vi "数字量输出配置.vi"() -> ()   [LabVIEW 2010] (continued)
              tunnel: [FALSE ("单选_第41路") TRUE ("单选_第41路")] -> w551
              frame False {
              }
              frame True {
              }
            }
            n6526 = local write "单选_第49路"(w551) -> ()
            n6527 = local write "单选_第50路"(w551) -> ()
            n6528 = local write "单选_第51路"(w551) -> ()
            n6529 = local write "单选_第52路"(w551) -> ()
            n6530 = local write "单选_第53路"(w551) -> ()
            n6531 = local write "单选_第54路"(w551) -> ()
            n6532 = local write "单选_第55路"(w551) -> ()
            n6533 = local write "单选_第56路"(w551) -> ()
            n6534 = local write "单选_第57路"(w551) -> ()
            n6535 = local write "单选_第58路"(w551) -> ()
            n6536 = local write "单选_第59路"(w551) -> ()
            n6537 = local write "单选_第60路"(w551) -> ()
            n6538 = local write "单选_第61路"(w551) -> ()
            n6539 = local write "单选_第62路"(w551) -> ()
            n6540 = local write "单选_第63路"(w551) -> ()
            n6541 = local write "单选_第64路"(w551) -> ()
          }
          event "btn_全选_5": Value Change {
            n6542 = event-data() -> ("NewVal"=w556:bool)  [unwired: 1 in, 4 out]
            n6543 = case shown="假" w556 {
              tunnel: [FALSE ("单选_第41路") TRUE ("单选_第41路")] -> w555
              frame False {
              }
              frame True {
              }
            }
            n6544 = local write "单选_第71路"(w555) -> ()
            n6545 = local write "单选_第79路"(w555) -> ()
            n6546 = local write "单选_第65路"(w555) -> ()
            n6547 = local write "单选_第66路"(w555) -> ()
            n6548 = local write "单选_第67路"(w555) -> ()
            n6549 = local write "单选_第68路"(w555) -> ()
            n6550 = local write "单选_第69路"(w555) -> ()
            n6551 = local write "单选_第70路"(w555) -> ()
            n6552 = local write "单选_第72路"(w555) -> ()
            n6553 = local write "单选_第73路"(w555) -> ()
            n6554 = local write "单选_第74路"(w555) -> ()
            n6555 = local write "单选_第75路"(w555) -> ()
            n6556 = local write "单选_第76路"(w555) -> ()
            n6557 = local write "单选_第77路"(w555) -> ()
            n6558 = local write "单选_第78路"(w555) -> ()
            n6559 = local write "单选_第80路"(w555) -> ()
          }
          event "btn_置1_1": Value Change {
            n6560 = event-data() -> ("NewVal"=w560:bool)  [unwired: 1 in, 4 out]
            n6561 = case shown="假" w560 {
              tunnel: [enum16{"0", "1"}."0" ("输入值_41") enum16{"0", "1"}."1" ("输入值_41")] -> w559
              frame False {
              }
              frame True {
              }
            }
            n6562 = local write "输入值_1"(w559) -> ()
            n6563 = local write "输入值_2"(w559) -> ()
            n6564 = local write "输入值_3"(w559) -> ()
            n6565 = local write "输入值_4"(w559) -> ()
            n6566 = local write "输入值_5"(w559) -> ()
            n6567 = local write "输入值_6"(w559) -> ()
            n6568 = local write "输入值_7"(w559) -> ()
            n6569 = local write "输入值_8"(w559) -> ()
            n6570 = local write "输入值_9"(w559) -> ()
            n6571 = local write "输入值_10"(w559) -> ()
            n6572 = local write "输入值_11"(w559) -> ()
            n6573 = local write "输入值_12"(w559) -> ()
            n6574 = local write "输入值_13"(w559) -> ()
            n6575 = local write "输入值_14"(w559) -> ()
            n6576 = local write "输入值_15"(w559) -> ()
            n6577 = local write "输入值_16"(w559) -> ()
          }
          event "btn_置1_2": Value Change {
            n6578 = event-data() -> ("NewVal"=w564:bool)  [unwired: 1 in, 4 out]
            n6579 = case shown="假" w564 {
              tunnel: [enum16{"0", "1"}."0" ("输入值_41") enum16{"0", "1"}."1" ("输入值_41")] -> w563
              frame False {
              }
              frame True {
              }
            }
            n6580 = local write "输入值_17"(w563) -> ()
            n6581 = local write "输入值_18"(w563) -> ()
            n6582 = local write "输入值_19"(w563) -> ()
            n6583 = local write "输入值_20"(w563) -> ()
            n6584 = local write "输入值_21"(w563) -> ()
            n6585 = local write "输入值_22"(w563) -> ()
            n6586 = local write "输入值_23"(w563) -> ()
            n6587 = local write "输入值_24"(w563) -> ()
            n6588 = local write "输入值_25"(w563) -> ()
            n6589 = local write "输入值_26"(w563) -> ()
            n6590 = local write "输入值_27"(w563) -> ()
            n6591 = local write "输入值_28"(w563) -> ()
            n6592 = local write "输入值_29"(w563) -> ()
            n6593 = local write "输入值_30"(w563) -> ()
            n6594 = local write "输入值_31"(w563) -> ()
            n6595 = local write "输入值_32"(w563) -> ()
          }
          event "btn_置1_3": Value Change {
            n6596 = event-data() -> ("NewVal"=w568:bool)  [unwired: 1 in, 4 out]
            n6597 = case shown="假" w568 {
              tunnel: [enum16{"0", "1"}."0" ("输入值_41") enum16{"0", "1"}."1" ("输入值_41")] -> w567
              frame False {
              }
              frame True {
              }
            }
            n6598 = local write "输入值_33"(w567) -> ()
            n6599 = local write "输入值_34"(w567) -> ()
            n6600 = local write "输入值_35"(w567) -> ()
            n6601 = local write "输入值_36"(w567) -> ()
            n6602 = local write "输入值_37"(w567) -> ()
            n6603 = local write "输入值_38"(w567) -> ()
            n6604 = local write "输入值_39"(w567) -> ()
            n6605 = local write "输入值_40"(w567) -> ()
            n6606 = local write "输入值_41"(w567) -> ()
            n6607 = local write "输入值_42"(w567) -> ()
            n6608 = local write "输入值_43"(w567) -> ()
            n6609 = local write "输入值_44"(w567) -> ()
            n6610 = local write "输入值_45"(w567) -> ()
            n6611 = local write "输入值_46"(w567) -> ()
            n6612 = local write "输入值_47"(w567) -> ()
            n6613 = local write "输入值_48"(w567) -> ()
          }
          event "btn_置1_4": Value Change {
            n6614 = event-data() -> ("NewVal"=w572:bool)  [unwired: 1 in, 4 out]
            n6615 = case shown="假" w572 {
              tunnel: [enum16{"0", "1"}."0" ("输入值_41") enum16{"0", "1"}."1" ("输入值_41")] -> w571
              frame False {
              }
              frame True {
              }
            }
            n6616 = local write "输入值_49"(w571) -> ()
            n6617 = local write "输入值_50"(w571) -> ()
            n6618 = local write "输入值_51"(w571) -> ()
            n6619 = local write "输入值_52"(w571) -> ()
            n6620 = local write "输入值_53"(w571) -> ()
            n6621 = local write "输入值_54"(w571) -> ()
            n6622 = local write "输入值_55"(w571) -> ()
            n6623 = local write "输入值_56"(w571) -> ()
            n6624 = local write "输入值_57"(w571) -> ()
            n6625 = local write "输入值_58"(w571) -> ()
            n6626 = local write "输入值_59"(w571) -> ()
            n6627 = local write "输入值_60"(w571) -> ()
            n6628 = local write "输入值_61"(w571) -> ()
            n6629 = local write "输入值_62"(w571) -> ()
            n6630 = local write "输入值_63"(w571) -> ()
            n6631 = local write "输入值_64"(w571) -> ()
          }
          event "btn_置1_5": Value Change {
            n6632 = event-data() -> ("NewVal"=w576:bool)  [unwired: 1 in, 4 out]
            n6633 = case shown="假" w576 {
              tunnel: [enum16{"0", "1"}."0" ("输入值_41") enum16{"0", "1"}."1" ("输入值_41")] -> w575
              frame False {
              }
              frame True {
              }
            }
            n6634 = local write "输入值_65"(w575) -> ()
            n6635 = local write "输入值_66"(w575) -> ()
            n6636 = local write "输入值_67"(w575) -> ()
            n6637 = local write "输入值_68"(w575) -> ()
            n6638 = local write "输入值_69"(w575) -> ()
            n6639 = local write "输入值_70"(w575) -> ()
            n6640 = local write "输入值_71"(w575) -> ()
            n6641 = local write "输入值_72"(w575) -> ()
            n6642 = local write "输入值_73"(w575) -> ()
            n6643 = local write "输入值_74"(w575) -> ()
            n6644 = local write "输入值_75"(w575) -> ()
            n6645 = local write "输入值_76"(w575) -> ()
            n6646 = local write "输入值_77"(w575) -> ()
            n6647 = local write "输入值_78"(w575) -> ()
            n6648 = local write "输入值_79"(w575) -> ()
            n6649 = local write "输入值_80"(w575) -> ()
          }
          event "btn_开始试验": Value Change {
            n6650 = event-data() -> ()  [unwired: 1 in, 5 out]
            n6651 = stacked-sequence {
              frame #0 {
                w580 = 0 ("同步_A1")
                n6652 = stacked-sequence {
                  tunnel: [w606 _ _ _ _] -> w602
                  tunnel: [w605 _ _ _ _] -> w586
                  tunnel: [_ w640 _ _ _] -> w600
                  tunnel: [_ w639 _ _ _] -> w585
                  tunnel: [_ _ w674 _ _] -> w598
                  tunnel: [_ _ w673 _ _] -> w584
                  tunnel: [_ _ _ w708 _] -> w596
                  tunnel: [_ _ _ w707 _] -> w583
                  tunnel: [_ _ _ _ w742] -> w594
                  tunnel: [_ _ _ _ w741] -> w582
                  frame #0 {
                    n6653 = local read "单选_第1路"() -> (w623:bool)
                    n6654 = local read "单选_第2路"() -> (w624:bool)
                    n6655 = local read "单选_第3路"() -> (w625:bool)
                    n6656 = local read "单选_第4路"() -> (w626:bool)
                    n6657 = local read "单选_第5路"() -> (w627:bool)
                    n6658 = local read "单选_第6路"() -> (w628:bool)
                    n6659 = local read "单选_第7路"() -> (w629:bool)
                    n6660 = local read "单选_第8路"() -> (w630:bool)
                    n6661 = local read "单选_第9路"() -> (w631:bool)
                    n6662 = local read "单选_第10路"() -> (w632:bool)
                    n6663 = local read "单选_第11路"() -> (w633:bool)
                    n6664 = local read "单选_第12路"() -> (w634:bool)
                    n6665 = local read "单选_第13路"() -> (w635:bool)
                    n6666 = local read "单选_第14路"() -> (w636:bool)
                    n6667 = local read "单选_第15路"() -> (w637:bool)
                    n6668 = local read "单选_第16路"() -> (w638:bool)
                    n6669 = local read "输入值_1"() -> (w607:enum16{"0", "1"})
                    n6670 = local read "输入值_2"() -> (w608:enum16{"0", "1"})
                    n6671 = local read "输入值_3"() -> (w609:enum16{"0", "1"})
                    n6672 = local read "输入值_4"() -> (w610:enum16{"0", "1"})
                    n6673 = local read "输入值_5"() -> (w611:enum16{"0", "1"})
                    n6674 = local read "输入值_6"() -> (w612:enum16{"0", "1"})
                    n6675 = local read "输入值_7"() -> (w613:enum16{"0", "1"})
                    n6676 = local read "输入值_8"() -> (w614:enum16{"0", "1"})
                    n6677 = local read "输入值_9"() -> (w615:enum16{"0", "1"})
                    n6678 = local read "输入值_10"() -> (w616:enum16{"0", "1"})
                    n6679 = local read "输入值_11"() -> (w617:enum16{"0", "1"})
                    n6680 = local read "输入值_12"() -> (w618:enum16{"0", "1"})
                    n6681 = local read "输入值_13"() -> (w619:enum16{"0", "1"})
                    n6682 = local read "输入值_14"() -> (w620:enum16{"0", "1"})
                    n6683 = local read "输入值_15"() -> (w621:enum16{"0", "1"})
                    n6684 = local read "输入值_16"() -> (w622:enum16{"0", "1"})
                    n6685 = Build Array(w623, w624, w625, w626, w627, w628, w629, w630, w631, w632, w633, w634, w635, w636, w637, w638) -> (w606:bool[])
                    n6686 = Build Array(w607, w608, w609, w610, w611, w612, w613, w614, w615, w616, w617, w618, w619, w620, w621, w622) -> (w605:enum16{"0", "1"}[])
                  }
                  frame #1 {
                    n6687 = local read "单选_第17路"() -> (w657:bool)
                    n6688 = local read "单选_第18路"() -> (w658:bool)
                    n6689 = local read "单选_第19路"() -> (w659:bool)
                    n6690 = local read "单选_第20路"() -> (w660:bool)
                    n6691 = local read "单选_第21路"() -> (w661:bool)
                    n6692 = local read "单选_第22路"() -> (w662:bool)
                    n6693 = local read "单选_第23路"() -> (w663:bool)
                    n6694 = local read "单选_第24路"() -> (w664:bool)
                    n6695 = local read "单选_第25路"() -> (w665:bool)
                    n6696 = local read "单选_第26路"() -> (w666:bool)
                    n6697 = local read "单选_第27路"() -> (w667:bool)
                    n6698 = local read "单选_第28路"() -> (w668:bool)
                    n6699 = local read "单选_第29路"() -> (w669:bool)
                    n6700 = local read "单选_第30路"() -> (w670:bool)
                    n6701 = local read "单选_第31路"() -> (w671:bool)
                    n6702 = local read "单选_第32路"() -> (w672:bool)
                    n6703 = local read "输入值_17"() -> (w641:enum16{"0", "1"})
                    n6704 = local read "输入值_18"() -> (w642:enum16{"0", "1"})
                    n6705 = local read "输入值_19"() -> (w643:enum16{"0", "1"})
                    n6706 = local read "输入值_20"() -> (w644:enum16{"0", "1"})
                    n6707 = local read "输入值_21"() -> (w645:enum16{"0", "1"})
                    n6708 = local read "输入值_22"() -> (w646:enum16{"0", "1"})
                    n6709 = local read "输入值_23"() -> (w647:enum16{"0", "1"})
                    n6710 = local read "输入值_24"() -> (w648:enum16{"0", "1"})
                    n6711 = local read "输入值_25"() -> (w649:enum16{"0", "1"})
                    n6712 = local read "输入值_26"() -> (w650:enum16{"0", "1"})
                    n6713 = local read "输入值_27"() -> (w651:enum16{"0", "1"})
                    n6714 = local read "输入值_28"() -> (w652:enum16{"0", "1"})
                    n6715 = local read "输入值_29"() -> (w653:enum16{"0", "1"})
                    n6716 = local read "输入值_30"() -> (w654:enum16{"0", "1"})
                    n6717 = local read "输入值_31"() -> (w655:enum16{"0", "1"})
                    n6718 = local read "输入值_32"() -> (w656:enum16{"0", "1"})
                    n6719 = Build Array(w657, w658, w659, w660, w661, w662, w663, w664, w665, w666, w667, w668, w669, w670, w671, w672) -> (w640:bool[])
                    n6720 = Build Array(w641, w642, w643, w644, w645, w646, w647, w648, w649, w650, w651, w652, w653, w654, w655, w656) -> (w639:enum16{"0", "1"}[])
                  }
                  frame #2 {
                    n6721 = local read "单选_第33路"() -> (w691:bool)
                    n6722 = local read "单选_第34路"() -> (w692:bool)
                    n6723 = local read "单选_第35路"() -> (w693:bool)
                    n6724 = local read "单选_第36路"() -> (w694:bool)
                    n6725 = local read "单选_第37路"() -> (w695:bool)
                    n6726 = local read "单选_第38路"() -> (w696:bool)
                    n6727 = local read "单选_第39路"() -> (w697:bool)
                    n6728 = local read "单选_第40路"() -> (w698:bool)
                    n6729 = local read "单选_第41路"() -> (w699:bool)
                    n6730 = local read "单选_第42路"() -> (w700:bool)
                    n6731 = local read "单选_第43路"() -> (w701:bool)
                    n6732 = local read "单选_第44路"() -> (w702:bool)
                    n6733 = local read "单选_第45路"() -> (w703:bool)
                    n6734 = local read "单选_第46路"() -> (w704:bool)
                    n6735 = local read "单选_第47路"() -> (w705:bool)
                    n6736 = local read "单选_第48路"() -> (w706:bool)
                    n6737 = local read "输入值_33"() -> (w675:enum16{"0", "1"})
                    n6738 = local read "输入值_34"() -> (w676:enum16{"0", "1"})
                    n6739 = local read "输入值_35"() -> (w677:enum16{"0", "1"})
                    n6740 = local read "输入值_36"() -> (w678:enum16{"0", "1"})
                    n6741 = local read "输入值_37"() -> (w679:enum16{"0", "1"})
                    n6742 = local read "输入值_38"() -> (w680:enum16{"0", "1"})
                    n6743 = local read "输入值_39"() -> (w681:enum16{"0", "1"})
                    n6744 = local read "输入值_40"() -> (w682:enum16{"0", "1"})
                    n6745 = local read "输入值_41"() -> (w683:enum16{"0", "1"})
                    n6746 = local read "输入值_42"() -> (w684:enum16{"0", "1"})
                    n6747 = local read "输入值_43"() -> (w685:enum16{"0", "1"})
                    n6748 = local read "输入值_44"() -> (w686:enum16{"0", "1"})
                    n6749 = local read "输入值_45"() -> (w687:enum16{"0", "1"})
                    n6750 = local read "输入值_46"() -> (w688:enum16{"0", "1"})
                    n6751 = local read "输入值_47"() -> (w689:enum16{"0", "1"})
                    n6752 = local read "输入值_48"() -> (w690:enum16{"0", "1"})
                    n6753 = Build Array(w675, w676, w677, w678, w679, w680, w681, w682, w683, w684, w685, w686, w687, w688, w689, w690) -> (w673:enum16{"0", "1"}[])
                    n6754 = Build Array(w691, w692, w693, w694, w695, w696, w697, w698, w699, w700, w701, w702, w703, w704, w705, w706) -> (w674:bool[])
                  }
                  frame #3 {
                    n6755 = local read "单选_第49路"() -> (w725:bool)
                    n6756 = local read "单选_第50路"() -> (w726:bool)
                    n6757 = local read "单选_第51路"() -> (w727:bool)
                    n6758 = local read "单选_第52路"() -> (w728:bool)
                    n6759 = local read "单选_第53路"() -> (w729:bool)
                    n6760 = local read "单选_第54路"() -> (w730:bool)
                    n6761 = local read "单选_第55路"() -> (w731:bool)
                    n6762 = local read "单选_第56路"() -> (w732:bool)
                    n6763 = local read "单选_第57路"() -> (w733:bool)
                    n6764 = local read "单选_第58路"() -> (w734:bool)
                    n6765 = local read "单选_第59路"() -> (w735:bool)
                    n6766 = local read "单选_第60路"() -> (w736:bool)
                    n6767 = local read "单选_第61路"() -> (w737:bool)
                    n6768 = local read "单选_第62路"() -> (w738:bool)
                    n6769 = local read "单选_第63路"() -> (w739:bool)
                    n6770 = local read "单选_第64路"() -> (w740:bool)
                    n6771 = local read "输入值_49"() -> (w709:enum16{"0", "1"})
                    n6772 = local read "输入值_50"() -> (w710:enum16{"0", "1"})
                    n6773 = local read "输入值_51"() -> (w711:enum16{"0", "1"})
                    n6774 = local read "输入值_52"() -> (w712:enum16{"0", "1"})
                    n6775 = local read "输入值_53"() -> (w713:enum16{"0", "1"})
                    n6776 = local read "输入值_54"() -> (w714:enum16{"0", "1"})
                    n6777 = local read "输入值_55"() -> (w715:enum16{"0", "1"})
                    n6778 = local read "输入值_56"() -> (w716:enum16{"0", "1"})
                    n6779 = local read "输入值_57"() -> (w717:enum16{"0", "1"})
                    n6780 = local read "输入值_58"() -> (w718:enum16{"0", "1"})
                    n6781 = local read "输入值_59"() -> (w719:enum16{"0", "1"})
                    n6782 = local read "输入值_60"() -> (w720:enum16{"0", "1"})
                    n6783 = local read "输入值_61"() -> (w721:enum16{"0", "1"})
                    n6784 = local read "输入值_62"() -> (w722:enum16{"0", "1"})
                    n6785 = local read "输入值_63"() -> (w723:enum16{"0", "1"})
                    n6786 = local read "输入值_64"() -> (w724:enum16{"0", "1"})
                    n6787 = Build Array(w725, w726, w727, w728, w729, w730, w731, w732, w733, w734, w735, w736, w737, w738, w739, w740) -> (w708:bool[])
                    n6788 = Build Array(w709, w710, w711, w712, w713, w714, w715, w716, w717, w718, w719, w720, w721, w722, w723, w724) -> (w707:enum16{"0", "1"}[])
                  }
                  frame #4 {
                    n6789 = local read "单选_第71路"() -> (w765:bool)
                    n6790 = local read "单选_第79路"() -> (w773:bool)
                    n6791 = local read "单选_第65路"() -> (w759:bool)
                    n6792 = local read "单选_第66路"() -> (w760:bool)
                    n6793 = local read "单选_第67路"() -> (w761:bool)
                    n6794 = local read "单选_第68路"() -> (w762:bool)
                    n6795 = local read "单选_第69路"() -> (w763:bool)
                    n6796 = local read "单选_第70路"() -> (w764:bool)
                    n6797 = local read "单选_第72路"() -> (w766:bool)
                    n6798 = local read "单选_第73路"() -> (w767:bool)
                    n6799 = local read "单选_第74路"() -> (w768:bool)
                    n6800 = local read "单选_第75路"() -> (w769:bool)
                    n6801 = local read "单选_第76路"() -> (w770:bool)
                    n6802 = local read "单选_第77路"() -> (w771:bool)
                    n6803 = local read "单选_第78路"() -> (w772:bool)
                    n6804 = local read "单选_第80路"() -> (w774:bool)
                    n6805 = local read "输入值_65"() -> (w743:enum16{"0", "1"})
                    n6806 = local read "输入值_66"() -> (w744:enum16{"0", "1"})
                    n6807 = local read "输入值_67"() -> (w745:enum16{"0", "1"})
                    n6808 = local read "输入值_68"() -> (w746:enum16{"0", "1"})
                    n6809 = local read "输入值_69"() -> (w747:enum16{"0", "1"})
                    n6810 = local read "输入值_70"() -> (w748:enum16{"0", "1"})
                    n6811 = local read "输入值_71"() -> (w749:enum16{"0", "1"})
                    n6812 = local read "输入值_72"() -> (w750:enum16{"0", "1"})
                    n6813 = local read "输入值_73"() -> (w751:enum16{"0", "1"})
                    n6814 = local read "输入值_74"() -> (w752:enum16{"0", "1"})
                    n6815 = local read "输入值_75"() -> (w753:enum16{"0", "1"})
                    n6816 = local read "输入值_76"() -> (w754:enum16{"0", "1"})
                    n6817 = local read "输入值_77"() -> (w755:enum16{"0", "1"})
                    n6818 = local read "输入值_78"() -> (w756:enum16{"0", "1"})
                    n6819 = local read "输入值_79"() -> (w757:enum16{"0", "1"})
                    n6820 = local read "输入值_80"() -> (w758:enum16{"0", "1"})
                    n6821 = Build Array(w743, w744, w745, w746, w747, w748, w749, w750, w751, w752, w753, w754, w755, w756, w757, w758) -> (w741:enum16{"0", "1"}[])
                    n6822 = Build Array(w759, w760, w761, w762, w763, w764, w765, w766, w767, w768, w769, w770, w771, w772, w773, w774) -> (w742:bool[])
                  }
                }
                n6823 = local read "数组_选择?"() -> (w604:bool[][])
                n6824 = local read "数组_输入值"() -> (w587:enum16{"0", "1"}[][])
                n6825 = Replace Array Subset(array=w604, new element #1=w602, index (row) #1=0 ("索引 (行)"), new element #2=w600, index (row) #2=1 ("索引 (行)"), new element #3=w598, index (row) #3=2 ("索引 (行)"), new element #4=w596, index (row) #4=3 ("索引 (行)"), new element #5=w594, index (row) #5=4 ("索引 (行)")) -> (w593:bool[][])  [unwired: 5 in]
                n6826 = local write "测试结论"("") -> ()
                n6827 = local write "同步_A1"(w580) -> ()
                n6828 = local write "同步_A2"(w580) -> ()
                n6829 = Replace Array Subset(array=w587, new element #1=w586, index (row) #1=0 ("索引 (行)"), new element #2=w585, index (row) #2=1 ("索引 (行)"), new element #3=w584, index (row) #3=2 ("索引 (行)"), new element #4=w583, index (row) #4=3 ("索引 (行)"), new element #5=w582, index (row) #5=4 ("索引 (行)")) -> (w581:enum16{"0", "1"}[][])  [unwired: 5 in]
                n6830 = local write "数组_输入值"(w581) -> ()
                n6831 = local write "数组_选择?"(w593) -> ()
              }
              frame #1 {
                w775 = cluster{u32, u32}[] [{9868950, 9868950}]
                n6832 = property on="light_1" class="Bool (严格)"("Colors [4]"=w775) -> ()  [unwired: 2 in, 2 out]
                n6833 = property on="light_2" class="Bool (严格)"("Colors [4]"=w775) -> ()  [unwired: 2 in, 2 out]
                n6834 = property on="light_3" class="Bool (严格)"("Colors [4]"=w775) -> ()  [unwired: 2 in, 2 out]
                n6835 = property on="light_4" class="Bool (严格)"("Colors [4]"=w775) -> ()  [unwired: 2 in, 2 out]
                n6836 = property on="light_5" class="Bool (严格)"("Colors [4]"=w775) -> ()  [unwired: 2 in, 2 out]
                n6837 = property on="light_6" class="Bool (严格)"("Colors [4]"=w775) -> ()  [unwired: 2 in, 2 out]
                n6838 = property on="light_7" class="Bool (严格)"("Colors [4]"=w775) -> ()  [unwired: 2 in, 2 out]
                n6839 = property on="light_8" class="Bool (严格)"("Colors [4]"=w775) -> ()  [unwired: 2 in, 2 out]
                n6840 = property on="light_9" class="Bool (严格)"("Colors [4]"=w775) -> ()  [unwired: 2 in, 2 out]
                n6841 = property on="light_10" class="Bool (严格)"("Colors [4]"=w775) -> ()  [unwired: 2 in, 2 out]
                n6842 = property on="light_11" class="Bool (严格)"("Colors [4]"=w775) -> ()  [unwired: 2 in, 2 out]
                n6843 = property on="light_12" class="Bool (严格)"("Colors [4]"=w775) -> ()  [unwired: 2 in, 2 out]
                n6844 = property on="light_13" class="Bool (严格)"("Colors [4]"=w775) -> ()  [unwired: 2 in, 2 out]
                n6845 = property on="light_14" class="Bool (严格)"("Colors [4]"=w775) -> ()  [unwired: 2 in, 2 out]
                n6846 = property on="light_15" class="Bool (严格)"("Colors [4]"=w775) -> ()  [unwired: 2 in, 2 out]
                n6847 = property on="light_16" class="Bool (严格)"("Colors [4]"=w775) -> ()  [unwired: 2 in, 2 out]
                n6848 = property on="light_17" class="Bool (严格)"("Colors [4]"=w775) -> ()  [unwired: 2 in, 2 out]
                n6849 = property on="light_18" class="Bool (严格)"("Colors [4]"=w775) -> ()  [unwired: 2 in, 2 out]
                n6850 = property on="light_19" class="Bool (严格)"("Colors [4]"=w775) -> ()  [unwired: 2 in, 2 out]
                n6851 = property on="light_20" class="Bool (严格)"("Colors [4]"=w775) -> ()  [unwired: 2 in, 2 out]
                n6852 = property on="light_21" class="Bool (严格)"("Colors [4]"=w775) -> ()  [unwired: 2 in, 2 out]
                n6853 = property on="light_22" class="Bool (严格)"("Colors [4]"=w775) -> ()  [unwired: 2 in, 2 out]
                n6854 = property on="light_23" class="Bool (严格)"("Colors [4]"=w775) -> ()  [unwired: 2 in, 2 out]
                n6855 = property on="light_24" class="Bool (严格)"("Colors [4]"=w775) -> ()  [unwired: 2 in, 2 out]
                n6856 = property on="light_25" class="Bool (严格)"("Colors [4]"=w775) -> ()  [unwired: 2 in, 2 out]
                n6857 = property on="light_26" class="Bool (严格)"("Colors [4]"=w775) -> ()  [unwired: 2 in, 2 out]
                n6858 = property on="light_27" class="Bool (严格)"("Colors [4]"=w775) -> ()  [unwired: 2 in, 2 out]
                n6859 = property on="light_28" class="Bool (严格)"("Colors [4]"=w775) -> ()  [unwired: 2 in, 2 out]
                n6860 = property on="light_29" class="Bool (严格)"("Colors [4]"=w775) -> ()  [unwired: 2 in, 2 out]
                n6861 = property on="light_30" class="Bool (严格)"("Colors [4]"=w775) -> ()  [unwired: 2 in, 2 out]
                n6862 = property on="light_31" class="Bool (严格)"("Colors [4]"=w775) -> ()  [unwired: 2 in, 2 out]
                n6863 = property on="light_32" class="Bool (严格)"("Colors [4]"=w775) -> ()  [unwired: 2 in, 2 out]
                n6864 = property on="light_33" class="Bool (严格)"("Colors [4]"=w775) -> ()  [unwired: 2 in, 2 out]
                n6865 = property on="light_34" class="Bool (严格)"("Colors [4]"=w775) -> ()  [unwired: 2 in, 2 out]
                n6866 = property on="light_35" class="Bool (严格)"("Colors [4]"=w775) -> ()  [unwired: 2 in, 2 out]
                n6867 = property on="light_36" class="Bool (严格)"("Colors [4]"=w775) -> ()  [unwired: 2 in, 2 out]
                n6868 = property on="light_37" class="Bool (严格)"("Colors [4]"=w775) -> ()  [unwired: 2 in, 2 out]
                n6869 = property on="light_38" class="Bool (严格)"("Colors [4]"=w775) -> ()  [unwired: 2 in, 2 out]
                n6870 = property on="light_39" class="Bool (严格)"("Colors [4]"=w775) -> ()  [unwired: 2 in, 2 out]
                n6871 = property on="light_40" class="Bool (严格)"("Colors [4]"=w775) -> ()  [unwired: 2 in, 2 out]
                n6872 = property on="light_41" class="Bool (严格)"("Colors [4]"=w775) -> ()  [unwired: 2 in, 2 out]
                n6873 = property on="light_42" class="Bool (严格)"("Colors [4]"=w775) -> ()  [unwired: 2 in, 2 out]
                n6874 = property on="light_43" class="Bool (严格)"("Colors [4]"=w775) -> ()  [unwired: 2 in, 2 out]
                n6875 = property on="light_44" class="Bool (严格)"("Colors [4]"=w775) -> ()  [unwired: 2 in, 2 out]
                n6876 = property on="light_45" class="Bool (严格)"("Colors [4]"=w775) -> ()  [unwired: 2 in, 2 out]
                n6877 = property on="light_46" class="Bool (严格)"("Colors [4]"=w775) -> ()  [unwired: 2 in, 2 out]
                n6878 = property on="light_47" class="Bool (严格)"("Colors [4]"=w775) -> ()  [unwired: 2 in, 2 out]
                n6879 = property on="light_48" class="Bool (严格)"("Colors [4]"=w775) -> ()  [unwired: 2 in, 2 out]
                n6880 = property on="light_49" class="Bool (严格)"("Colors [4]"=w775) -> ()  [unwired: 2 in, 2 out]
                n6881 = property on="light_50" class="Bool (严格)"("Colors [4]"=w775) -> ()  [unwired: 2 in, 2 out]
                n6882 = property on="light_51" class="Bool (严格)"("Colors [4]"=w775) -> ()  [unwired: 2 in, 2 out]
                n6883 = property on="light_52" class="Bool (严格)"("Colors [4]"=w775) -> ()  [unwired: 2 in, 2 out]
                n6884 = property on="light_53" class="Bool (严格)"("Colors [4]"=w775) -> ()  [unwired: 2 in, 2 out]
                n6885 = property on="light_54" class="Bool (严格)"("Colors [4]"=w775) -> ()  [unwired: 2 in, 2 out]
                n6886 = property on="light_55" class="Bool (严格)"("Colors [4]"=w775) -> ()  [unwired: 2 in, 2 out]
                n6887 = property on="light_56" class="Bool (严格)"("Colors [4]"=w775) -> ()  [unwired: 2 in, 2 out]
                n6888 = property on="light_57" class="Bool (严格)"("Colors [4]"=w775) -> ()  [unwired: 2 in, 2 out]
                n6889 = property on="light_58" class="Bool (严格)"("Colors [4]"=w775) -> ()  [unwired: 2 in, 2 out]
                n6890 = property on="light_59" class="Bool (严格)"("Colors [4]"=w775) -> ()  [unwired: 2 in, 2 out]
                n6891 = property on="light_60" class="Bool (严格)"("Colors [4]"=w775) -> ()  [unwired: 2 in, 2 out]
                n6892 = property on="light_61" class="Bool (严格)"("Colors [4]"=w775) -> ()  [unwired: 2 in, 2 out]
                n6893 = property on="light_62" class="Bool (严格)"("Colors [4]"=w775) -> ()  [unwired: 2 in, 2 out]
                n6894 = property on="light_63" class="Bool (严格)"("Colors [4]"=w775) -> ()  [unwired: 2 in, 2 out]
                n6895 = property on="light_64" class="Bool (严格)"("Colors [4]"=w775) -> ()  [unwired: 2 in, 2 out]
                n6896 = property on="light_65" class="Bool (严格)"("Colors [4]"=w775) -> ()  [unwired: 2 in, 2 out]
                n6897 = property on="light_66" class="Bool (严格)"("Colors [4]"=w775) -> ()  [unwired: 2 in, 2 out]
                n6898 = property on="light_67" class="Bool (严格)"("Colors [4]"=w775) -> ()  [unwired: 2 in, 2 out]
                n6899 = property on="light_68" class="Bool (严格)"("Colors [4]"=w775) -> ()  [unwired: 2 in, 2 out]
                n6900 = property on="light_69" class="Bool (严格)"("Colors [4]"=w775) -> ()  [unwired: 2 in, 2 out]
                n6901 = property on="light_70" class="Bool (严格)"("Colors [4]"=w775) -> ()  [unwired: 2 in, 2 out]
                n6902 = property on="light_71" class="Bool (严格)"("Colors [4]"=w775) -> ()  [unwired: 2 in, 2 out]
                n6903 = property on="light_72" class="Bool (严格)"("Colors [4]"=w775) -> ()  [unwired: 2 in, 2 out]
                n6904 = property on="light_73" class="Bool (严格)"("Colors [4]"=w775) -> ()  [unwired: 2 in, 2 out]
                n6905 = property on="light_74" class="Bool (严格)"("Colors [4]"=w775) -> ()  [unwired: 2 in, 2 out]
                n6906 = property on="light_75" class="Bool (严格)"("Colors [4]"=w775) -> ()  [unwired: 2 in, 2 out]
                n6907 = property on="light_76" class="Bool (严格)"("Colors [4]"=w775) -> ()  [unwired: 2 in, 2 out]
                n6908 = property on="light_77" class="Bool (严格)"("Colors [4]"=w775) -> ()  [unwired: 2 in, 2 out]
                n6909 = property on="light_78" class="Bool (严格)"("Colors [4]"=w775) -> ()  [unwired: 2 in, 2 out]
                n6910 = property on="light_79" class="Bool (严格)"("Colors [4]"=w775) -> ()  [unwired: 2 in, 2 out]
                n6911 = property on="light_80" class="Bool (严格)"("Colors [4]"=w775) -> ()  [unwired: 2 in, 2 out]
                n6912 = Initialize Array("", 16 ("维数大小"), 4 ("维数大小")) -> (w779:string[][])
                n6913 = local write "D_IN_1"(w779) -> ()
                n6914 = local write "D_IN_2"(w779) -> ()
                n6915 = local write "D_IN_3"(w779) -> ()
                n6916 = local write "D_IN_4"(w779) -> ()
                n6917 = local write "D_IN_5"(w779) -> ()
              }
              frame #2 {
                n6918 = local read "保持输出"() -> (w780:bool)
                n6919 = case shown="假" w780 {
                  frame False {
                    n6920 = property on="保持输出" class="Bool (严格)"("DisabledEnum"=T1."Disabled and Grayed Out" ("禁用")) -> ()  [unwired: 2 in, 2 out]
                  }
                  frame True {
                    n6921 = local read "数组_选择?"() -> (w782:bool[][])
                    n6922 = for {
                      tunnel: w782 -> [w786] mode=indexing
                      i -> [w784]
                      stop <- w783 stop-if-true
                      n6923 = Or Array Elements(Boolean array=w786) -> (logical OR=w785:bool)
                      n6924 = case shown="真" w785 {
                        tunnel: w784 -> [_ w788]
                        tunnel: [FALSE TRUE] -> w783
                        frame False {
                        }
                        frame True {
                          n6925 = local write "同步_A1"(w788) -> ()
                          n6926 = Increment(x=w788) -> (x+1=w792:i32)
                          n6927 = Format Into String(format string="保持第%d组数据输出" ("格式字符串"), w792) -> (resulting string=w791:string)  [unwired: 2 in, 1 out]
                          n6928 = call "显示对话框信息5"("Message"=w791) -> ("是"=w789:bool)  [unwired: 9 in, 1 out]
                          n6929 = case shown="真" w789 {
                            tunnel: w788 -> [_ w794]
                            frame False {
                            }
                            frame True {
                              n6930 = stacked-sequence {
                                tunnel: w794 -> [w795 _]
                                frame #0 {
                                n6931 = for {
                                N: 5 -> [_]
                                tunnel: w795 -> [w798]
                                i -> [w797]
                                n6932 = Not Equal?(x=w798, y=w797) -> (x != y?=w799:bool)
                                n6933 = case shown="真" w799 {
                                tunnel: w797 -> [_ w803]
                                frame False {
                                }
                                frame True {
                                n6934 = local read "数组_选择?"() -> (w805:bool[][])
                                n6935 = Initialize Array(FALSE, 16 ("维数大小")) -> (w800:bool[])
                                n6936 = Replace Array Subset(array=w805, new element=w800, index (row)=w803) -> (w804:bool[][])  [unwired: 1 in]
                                n6937 = local write "数组_选择?"(w804) -> ()
                                }
                                }
                                }
                                }
                                frame #1 {
                                n6938 = property on="btn_开始试验" class="Bool"("DisabledEnum"=T1."Disabled and Grayed Out" ("禁用")) -> ()  [unwired: 2 in, 2 out]
                                }
                              }
                            }
                          }
                          n6939 = local write "保持输出"(w789) -> ()
                        }
                      }
                    }
                  }
                }
              }
              frame #3 {
                n6940 = local read "数组_选择?"() -> (w808:bool[][])
                n6941 = Or Array Elements(Boolean array=w808) -> (logical OR=w807:bool)
                n6942 = case shown="真" w807 {
                  frame False {
                    n6943 = call "显示对话框信息"("Message"="请选择数字量输入路数") -> ()  [unwired: 9 in, 2 out]
                  }
                  frame True {
                    w811 = "DOStart" ("名称（未命名）")
                    n6944 = Obtain Notifier(name (unnamed)=w811, notification data type=w811) -> (notifier out=w810:refnum<notifier>)  [unwired: 2 in, 2 out]
                    n6945 = Send Notification(notification="DOutput" ("通知"), notifier=w810) -> ()  [unwired: 1 in, 2 out]
                  }
                }
              }
            }
          }
          event "保持输出": Value Change {
            n6946 = event-data() -> ()  [unwired: 1 in, 5 out]
            n6947 = property on="btn_开始试验" class="Bool"("DisabledEnum"=T1."Enabled" ("禁用")) -> ()  [unwired: 2 in, 2 out]
          }
          event "btn_全选": Value Change {
            w814 = TRUE ("单选_第41路")
            n6948 = event-data() -> ()  [unwired: 1 in, 5 out]
            n6949 = local write "单选_第1路"(w814) -> ()
            n6950 = local write "单选_第2路"(w814) -> ()
            n6951 = local write "单选_第3路"(w814) -> ()
            n6952 = local write "单选_第4路"(w814) -> ()
            n6953 = local write "单选_第5路"(w814) -> ()
            n6954 = local write "单选_第6路"(w814) -> ()
            n6955 = local write "单选_第7路"(w814) -> ()
            n6956 = local write "单选_第8路"(w814) -> ()
            n6957 = local write "单选_第9路"(w814) -> ()
            n6958 = local write "单选_第10路"(w814) -> ()
            n6959 = local write "单选_第11路"(w814) -> ()
            n6960 = local write "单选_第12路"(w814) -> ()
            n6961 = local write "单选_第13路"(w814) -> ()
            n6962 = local write "单选_第14路"(w814) -> ()
            n6963 = local write "单选_第15路"(w814) -> ()
            n6964 = local write "单选_第16路"(w814) -> ()
            n6965 = local write "单选_第17路"(w814) -> ()
            n6966 = local write "单选_第18路"(w814) -> ()
            n6967 = local write "单选_第19路"(w814) -> ()
            n6968 = local write "单选_第20路"(w814) -> ()
            n6969 = local write "单选_第21路"(w814) -> ()
            n6970 = local write "单选_第22路"(w814) -> ()
            n6971 = local write "单选_第23路"(w814) -> ()
            n6972 = local write "单选_第24路"(w814) -> ()
            n6973 = local write "单选_第25路"(w814) -> ()
            n6974 = local write "单选_第26路"(w814) -> ()
            n6975 = local write "单选_第27路"(w814) -> ()
            n6976 = local write "单选_第28路"(w814) -> ()
            n6977 = local write "单选_第29路"(w814) -> ()
            n6978 = local write "单选_第30路"(w814) -> ()
            n6979 = local write "单选_第31路"(w814) -> ()
            n6980 = local write "单选_第32路"(w814) -> ()
            n6981 = local write "单选_第33路"(w814) -> ()
            n6982 = local write "单选_第34路"(w814) -> ()
            n6983 = local write "单选_第35路"(w814) -> ()
            n6984 = local write "单选_第36路"(w814) -> ()
            n6985 = local write "单选_第37路"(w814) -> ()
            n6986 = local write "单选_第38路"(w814) -> ()
            n6987 = local write "单选_第39路"(w814) -> ()
            n6988 = local write "单选_第40路"(w814) -> ()
            n6989 = local write "单选_第41路"(w814) -> ()
            n6990 = local write "单选_第42路"(w814) -> ()
            n6991 = local write "单选_第43路"(w814) -> ()
            n6992 = local write "单选_第44路"(w814) -> ()
            n6993 = local write "单选_第45路"(w814) -> ()
            n6994 = local write "单选_第46路"(w814) -> ()
            n6995 = local write "单选_第47路"(w814) -> ()
            n6996 = local write "单选_第48路"(w814) -> ()
            n6997 = local write "单选_第49路"(w814) -> ()
            n6998 = local write "单选_第50路"(w814) -> ()
            n6999 = local write "单选_第51路"(w814) -> ()
            n7000 = local write "单选_第52路"(w814) -> ()
            n7001 = local write "单选_第53路"(w814) -> ()
            n7002 = local write "单选_第54路"(w814) -> ()
            n7003 = local write "单选_第55路"(w814) -> ()
            n7004 = local write "单选_第56路"(w814) -> ()
            n7005 = local write "单选_第57路"(w814) -> ()
            n7006 = local write "单选_第58路"(w814) -> ()
            n7007 = local write "单选_第59路"(w814) -> ()
            n7008 = local write "单选_第60路"(w814) -> ()
            n7009 = local write "单选_第61路"(w814) -> ()
            n7010 = local write "单选_第62路"(w814) -> ()
            n7011 = local write "单选_第63路"(w814) -> ()
            n7012 = local write "单选_第64路"(w814) -> ()
            n7013 = local write "单选_第71路"(w814) -> ()
            n7014 = local write "单选_第79路"(w814) -> ()
            n7015 = local write "单选_第65路"(w814) -> ()
            n7016 = local write "单选_第66路"(w814) -> ()
            n7017 = local write "单选_第67路"(w814) -> ()
            n7018 = local write "单选_第68路"(w814) -> ()
            n7019 = local write "单选_第69路"(w814) -> ()
            n7020 = local write "单选_第70路"(w814) -> ()
            n7021 = local write "单选_第72路"(w814) -> ()
            n7022 = local write "单选_第73路"(w814) -> ()
            n7023 = local write "单选_第74路"(w814) -> ()
            n7024 = local write "单选_第75路"(w814) -> ()
            n7025 = local write "单选_第76路"(w814) -> ()
            n7026 = local write "单选_第77路"(w814) -> ()
            n7027 = local write "单选_第78路"(w814) -> ()
            n7028 = local write "单选_第80路"(w814) -> ()
          }
          event "btn_反选": Value Change {
            n7029 = event-data() -> ()  [unwired: 1 in, 5 out]
            n7030 = local read "单选_第1路"() -> (w974:bool)
            n7031 = local read "单选_第2路"() -> (w972:bool)
            n7032 = local read "单选_第3路"() -> (w970:bool)
            n7033 = local read "单选_第4路"() -> (w968:bool)
            n7034 = local read "单选_第5路"() -> (w966:bool)
            n7035 = local read "单选_第6路"() -> (w964:bool)
            n7036 = local read "单选_第7路"() -> (w963:bool)
            n7037 = local read "单选_第8路"() -> (w962:bool)
            n7038 = local read "单选_第9路"() -> (w961:bool)
            n7039 = local read "单选_第10路"() -> (w960:bool)
            n7040 = local read "单选_第11路"() -> (w959:bool)
            n7041 = local read "单选_第12路"() -> (w958:bool)
            n7042 = local read "单选_第13路"() -> (w957:bool)
            n7043 = local read "单选_第14路"() -> (w956:bool)
            n7044 = local read "单选_第15路"() -> (w955:bool)
            n7045 = local read "单选_第16路"() -> (w954:bool)
            n7046 = local read "单选_第17路"() -> (w953:bool)
            n7047 = local read "单选_第18路"() -> (w952:bool)
            n7048 = local read "单选_第19路"() -> (w951:bool)
            n7049 = local read "单选_第20路"() -> (w950:bool)
            n7050 = local read "单选_第21路"() -> (w949:bool)
            n7051 = local read "单选_第22路"() -> (w948:bool)
            n7052 = local read "单选_第23路"() -> (w947:bool)
            n7053 = local read "单选_第24路"() -> (w946:bool)
            n7054 = local read "单选_第25路"() -> (w945:bool)
            n7055 = local read "单选_第26路"() -> (w944:bool)
            n7056 = local read "单选_第27路"() -> (w943:bool)
            n7057 = local read "单选_第28路"() -> (w942:bool)
            n7058 = local read "单选_第29路"() -> (w941:bool)
            n7059 = local read "单选_第30路"() -> (w940:bool)
            n7060 = local read "单选_第31路"() -> (w939:bool)
            n7061 = local read "单选_第32路"() -> (w938:bool)
            n7062 = local read "单选_第33路"() -> (w937:bool)
            n7063 = local read "单选_第34路"() -> (w936:bool)
            n7064 = local read "单选_第35路"() -> (w935:bool)
            n7065 = local read "单选_第36路"() -> (w934:bool)
            n7066 = local read "单选_第37路"() -> (w933:bool)
            n7067 = local read "单选_第38路"() -> (w932:bool)
            n7068 = local read "单选_第39路"() -> (w931:bool)
            n7069 = local read "单选_第40路"() -> (w930:bool)
            n7070 = Not(x=w974) -> (.not. x?=w973:bool)
            n7071 = Not(x=w972) -> (.not. x?=w971:bool)
            n7072 = Not(x=w970) -> (.not. x?=w969:bool)
            n7073 = Not(x=w968) -> (.not. x?=w967:bool)
            n7074 = Not(x=w966) -> (.not. x?=w965:bool)
            n7075 = Not(x=w964) -> (.not. x?=w929:bool)
            n7076 = Not(x=w963) -> (.not. x?=w928:bool)
            n7077 = Not(x=w962) -> (.not. x?=w927:bool)
            n7078 = Not(x=w961) -> (.not. x?=w926:bool)
            n7079 = Not(x=w960) -> (.not. x?=w925:bool)
            n7080 = Not(x=w959) -> (.not. x?=w924:bool)
            n7081 = Not(x=w958) -> (.not. x?=w923:bool)
            n7082 = Not(x=w957) -> (.not. x?=w922:bool)
            n7083 = Not(x=w956) -> (.not. x?=w921:bool)
            n7084 = Not(x=w955) -> (.not. x?=w920:bool)
            n7085 = Not(x=w954) -> (.not. x?=w919:bool)
            n7086 = Not(x=w953) -> (.not. x?=w918:bool)
            n7087 = Not(x=w952) -> (.not. x?=w917:bool)
            n7088 = Not(x=w951) -> (.not. x?=w916:bool)
            n7089 = Not(x=w950) -> (.not. x?=w915:bool)
            n7090 = Not(x=w949) -> (.not. x?=w914:bool)
            n7091 = Not(x=w948) -> (.not. x?=w913:bool)
            n7092 = Not(x=w947) -> (.not. x?=w912:bool)
            n7093 = Not(x=w946) -> (.not. x?=w911:bool)
            n7094 = Not(x=w945) -> (.not. x?=w910:bool)
            n7095 = Not(x=w944) -> (.not. x?=w909:bool)
            n7096 = Not(x=w943) -> (.not. x?=w908:bool)
            n7097 = Not(x=w942) -> (.not. x?=w907:bool)
            n7098 = Not(x=w941) -> (.not. x?=w906:bool)
            n7099 = Not(x=w940) -> (.not. x?=w905:bool)
            n7100 = Not(x=w939) -> (.not. x?=w904:bool)
            n7101 = Not(x=w938) -> (.not. x?=w903:bool)
            n7102 = Not(x=w937) -> (.not. x?=w902:bool)
            n7103 = Not(x=w936) -> (.not. x?=w901:bool)
            n7104 = Not(x=w935) -> (.not. x?=w900:bool)
            n7105 = Not(x=w934) -> (.not. x?=w899:bool)
            n7106 = Not(x=w933) -> (.not. x?=w898:bool)
            n7107 = Not(x=w932) -> (.not. x?=w897:bool)
            n7108 = Not(x=w931) -> (.not. x?=w896:bool)
            n7109 = Not(x=w930) -> (.not. x?=w895:bool)
            n7110 = local write "单选_第1路"(w973) -> ()
            n7111 = local write "单选_第2路"(w971) -> ()
            n7112 = local write "单选_第3路"(w969) -> ()
            n7113 = local write "单选_第4路"(w967) -> ()
            n7114 = local write "单选_第5路"(w965) -> ()
            n7115 = local write "单选_第6路"(w929) -> ()
            n7116 = local write "单选_第7路"(w928) -> ()
            n7117 = local write "单选_第8路"(w927) -> ()
            n7118 = local write "单选_第9路"(w926) -> ()
            n7119 = local write "单选_第10路"(w925) -> ()
            n7120 = local write "单选_第11路"(w924) -> ()
            n7121 = local write "单选_第12路"(w923) -> ()
            n7122 = local write "单选_第13路"(w922) -> ()
            n7123 = local write "单选_第14路"(w921) -> ()
            n7124 = local write "单选_第15路"(w920) -> ()
            n7125 = local write "单选_第16路"(w919) -> ()
            n7126 = local write "单选_第17路"(w918) -> ()
            n7127 = local write "单选_第18路"(w917) -> ()
            n7128 = local write "单选_第19路"(w916) -> ()
            n7129 = local write "单选_第20路"(w915) -> ()
            n7130 = local write "单选_第21路"(w914) -> ()
            n7131 = local write "单选_第22路"(w913) -> ()
            n7132 = local write "单选_第23路"(w912) -> ()
            n7133 = local write "单选_第24路"(w911) -> ()
            n7134 = local write "单选_第25路"(w910) -> ()
            n7135 = local write "单选_第26路"(w909) -> ()
            n7136 = local write "单选_第27路"(w908) -> ()
            n7137 = local write "单选_第28路"(w907) -> ()
            n7138 = local write "单选_第29路"(w906) -> ()
            n7139 = local write "单选_第30路"(w905) -> ()
            n7140 = local write "单选_第31路"(w904) -> ()
            n7141 = local write "单选_第32路"(w903) -> ()
            n7142 = local write "单选_第33路"(w902) -> ()
            n7143 = local write "单选_第34路"(w901) -> ()
            n7144 = local write "单选_第35路"(w900) -> ()
            n7145 = local write "单选_第36路"(w899) -> ()
            n7146 = local write "单选_第37路"(w898) -> ()
            n7147 = local write "单选_第38路"(w897) -> ()
            n7148 = local write "单选_第39路"(w896) -> ()
            n7149 = local write "单选_第40路"(w895) -> ()
            n7150 = local read "单选_第71路"() -> (w864:bool)
            n7151 = local read "单选_第79路"() -> (w856:bool)
            n7152 = local read "单选_第41路"() -> (w894:bool)
            n7153 = local read "单选_第42路"() -> (w893:bool)
            n7154 = local read "单选_第43路"() -> (w892:bool)
            n7155 = local read "单选_第44路"() -> (w891:bool)
            n7156 = local read "单选_第45路"() -> (w890:bool)
            n7157 = local read "单选_第46路"() -> (w889:bool)
            n7158 = local read "单选_第47路"() -> (w888:bool)
            n7159 = local read "单选_第48路"() -> (w887:bool)
            n7160 = local read "单选_第49路"() -> (w886:bool)
            n7161 = local read "单选_第50路"() -> (w885:bool)
            n7162 = local read "单选_第51路"() -> (w884:bool)
            n7163 = local read "单选_第52路"() -> (w883:bool)
            n7164 = local read "单选_第53路"() -> (w882:bool)
            n7165 = local read "单选_第54路"() -> (w881:bool)
            n7166 = local read "单选_第55路"() -> (w880:bool)
            n7167 = local read "单选_第56路"() -> (w879:bool)
            n7168 = local read "单选_第57路"() -> (w878:bool)
            n7169 = local read "单选_第58路"() -> (w877:bool)
            n7170 = local read "单选_第59路"() -> (w876:bool)
            n7171 = local read "单选_第60路"() -> (w875:bool)
            n7172 = local read "单选_第61路"() -> (w874:bool)
            n7173 = local read "单选_第62路"() -> (w873:bool)
            n7174 = local read "单选_第63路"() -> (w872:bool)
            n7175 = local read "单选_第64路"() -> (w871:bool)
            n7176 = local read "单选_第65路"() -> (w870:bool)
            n7177 = local read "单选_第66路"() -> (w869:bool)
            n7178 = local read "单选_第67路"() -> (w868:bool)
            n7179 = local read "单选_第68路"() -> (w867:bool)
            n7180 = local read "单选_第69路"() -> (w866:bool)
            n7181 = local read "单选_第70路"() -> (w865:bool)
            n7182 = local read "单选_第72路"() -> (w863:bool)
            n7183 = local read "单选_第73路"() -> (w862:bool)
            n7184 = local read "单选_第74路"() -> (w861:bool)
            n7185 = local read "单选_第75路"() -> (w860:bool)
            n7186 = local read "单选_第76路"() -> (w859:bool)
            n7187 = local read "单选_第77路"() -> (w858:bool)
            n7188 = local read "单选_第78路"() -> (w857:bool)
            n7189 = local read "单选_第80路"() -> (w855:bool)
            n7190 = Not(x=w894) -> (.not. x?=w854:bool)
            n7191 = Not(x=w893) -> (.not. x?=w853:bool)
            n7192 = Not(x=w892) -> (.not. x?=w852:bool)
            n7193 = Not(x=w891) -> (.not. x?=w851:bool)
            n7194 = Not(x=w890) -> (.not. x?=w850:bool)
            n7195 = Not(x=w889) -> (.not. x?=w849:bool)
            n7196 = Not(x=w888) -> (.not. x?=w848:bool)
            n7197 = Not(x=w887) -> (.not. x?=w847:bool)
            n7198 = Not(x=w886) -> (.not. x?=w846:bool)
            n7199 = Not(x=w885) -> (.not. x?=w845:bool)
            n7200 = Not(x=w884) -> (.not. x?=w844:bool)
            n7201 = Not(x=w883) -> (.not. x?=w843:bool)
            n7202 = Not(x=w882) -> (.not. x?=w842:bool)
            n7203 = Not(x=w881) -> (.not. x?=w841:bool)
            n7204 = Not(x=w880) -> (.not. x?=w840:bool)
            n7205 = Not(x=w879) -> (.not. x?=w839:bool)
            n7206 = Not(x=w878) -> (.not. x?=w838:bool)
            n7207 = Not(x=w877) -> (.not. x?=w837:bool)
            n7208 = Not(x=w876) -> (.not. x?=w836:bool)
            n7209 = Not(x=w875) -> (.not. x?=w835:bool)
            n7210 = Not(x=w874) -> (.not. x?=w834:bool)
            n7211 = Not(x=w873) -> (.not. x?=w833:bool)
            n7212 = Not(x=w872) -> (.not. x?=w832:bool)
            n7213 = Not(x=w871) -> (.not. x?=w831:bool)
            n7214 = Not(x=w870) -> (.not. x?=w830:bool)
            n7215 = Not(x=w869) -> (.not. x?=w829:bool)
            n7216 = Not(x=w868) -> (.not. x?=w828:bool)
            n7217 = Not(x=w867) -> (.not. x?=w827:bool)
            n7218 = Not(x=w866) -> (.not. x?=w826:bool)
            n7219 = Not(x=w865) -> (.not. x?=w825:bool)
            n7220 = Not(x=w864) -> (.not. x?=w824:bool)
            n7221 = Not(x=w863) -> (.not. x?=w823:bool)
            n7222 = Not(x=w862) -> (.not. x?=w822:bool)
            n7223 = Not(x=w861) -> (.not. x?=w821:bool)
            n7224 = Not(x=w860) -> (.not. x?=w820:bool)
            n7225 = Not(x=w859) -> (.not. x?=w819:bool)
            n7226 = Not(x=w858) -> (.not. x?=w818:bool)
            n7227 = Not(x=w857) -> (.not. x?=w817:bool)
            n7228 = Not(x=w856) -> (.not. x?=w816:bool)
            n7229 = Not(x=w855) -> (.not. x?=w815:bool)
            n7230 = local write "单选_第71路"(w824) -> ()
            n7231 = local write "单选_第79路"(w816) -> ()
            n7232 = local write "单选_第41路"(w854) -> ()
            n7233 = local write "单选_第42路"(w853) -> ()
            n7234 = local write "单选_第43路"(w852) -> ()
            n7235 = local write "单选_第44路"(w851) -> ()
            n7236 = local write "单选_第45路"(w850) -> ()
            n7237 = local write "单选_第46路"(w849) -> ()
            n7238 = local write "单选_第47路"(w848) -> ()
            n7239 = local write "单选_第48路"(w847) -> ()
            n7240 = local write "单选_第49路"(w846) -> ()
            n7241 = local write "单选_第50路"(w845) -> ()
            n7242 = local write "单选_第51路"(w844) -> ()
            n7243 = local write "单选_第52路"(w843) -> ()
            n7244 = local write "单选_第53路"(w842) -> ()
            n7245 = local write "单选_第54路"(w841) -> ()
            n7246 = local write "单选_第55路"(w840) -> ()
            n7247 = local write "单选_第56路"(w839) -> ()
            n7248 = local write "单选_第57路"(w838) -> ()
            n7249 = local write "单选_第58路"(w837) -> ()
            n7250 = local write "单选_第59路"(w836) -> ()
            n7251 = local write "单选_第60路"(w835) -> ()
            n7252 = local write "单选_第61路"(w834) -> ()
            n7253 = local write "单选_第62路"(w833) -> ()
            n7254 = local write "单选_第63路"(w832) -> ()
            n7255 = local write "单选_第64路"(w831) -> ()
            n7256 = local write "单选_第65路"(w830) -> ()
            n7257 = local write "单选_第66路"(w829) -> ()
            n7258 = local write "单选_第67路"(w828) -> ()
            n7259 = local write "单选_第68路"(w827) -> ()
            n7260 = local write "单选_第69路"(w826) -> ()
            n7261 = local write "单选_第70路"(w825) -> ()
            n7262 = local write "单选_第72路"(w823) -> ()
            n7263 = local write "单选_第73路"(w822) -> ()
            n7264 = local write "单选_第74路"(w821) -> ()
            n7265 = local write "单选_第75路"(w820) -> ()
            n7266 = local write "单选_第76路"(w819) -> ()
            n7267 = local write "单选_第77路"(w818) -> ()
            n7268 = local write "单选_第78路"(w817) -> ()
            n7269 = local write "单选_第80路"(w815) -> ()
          }
          event "btn_置1": Value Change {
            w975 = enum16{"0", "1"}."1" ("输入值_41")
            n7270 = event-data() -> ()  [unwired: 1 in, 5 out]
            n7271 = local write "输入值_1"(w975) -> ()
            n7272 = local write "输入值_2"(w975) -> ()
            n7273 = local write "输入值_3"(w975) -> ()
            n7274 = local write "输入值_4"(w975) -> ()
            n7275 = local write "输入值_5"(w975) -> ()
            n7276 = local write "输入值_6"(w975) -> ()
            n7277 = local write "输入值_7"(w975) -> ()
            n7278 = local write "输入值_8"(w975) -> ()
            n7279 = local write "输入值_9"(w975) -> ()
            n7280 = local write "输入值_10"(w975) -> ()
            n7281 = local write "输入值_11"(w975) -> ()
            n7282 = local write "输入值_12"(w975) -> ()
            n7283 = local write "输入值_13"(w975) -> ()
            n7284 = local write "输入值_14"(w975) -> ()
            n7285 = local write "输入值_15"(w975) -> ()
            n7286 = local write "输入值_16"(w975) -> ()
            n7287 = local write "输入值_17"(w975) -> ()
            n7288 = local write "输入值_18"(w975) -> ()
            n7289 = local write "输入值_19"(w975) -> ()
            n7290 = local write "输入值_20"(w975) -> ()
            n7291 = local write "输入值_21"(w975) -> ()
            n7292 = local write "输入值_22"(w975) -> ()
            n7293 = local write "输入值_23"(w975) -> ()
            n7294 = local write "输入值_24"(w975) -> ()
            n7295 = local write "输入值_25"(w975) -> ()
